vi "DosageCtl.vi"(0 "setpoint volume flow [l/min]":sgl, 1 "pump":bool, 2 "value speed [%]":u8, 3 "shiftReg int":u64, 4 "shiftReg dbl":dbl, 5 "error in (no error)":errorcluster, 6 "setpoint volume [l]":sgl, 7 "value volume flow [l/min]":dbl, 8 "enable":bool, 9 "value volume [dl]":u64, 10 "Actual Start [f]":i64) -> (12 "pump":bool, 14 "speed [%]":dbl, 15 "shiftReg int":u64, 16 "shiftreg dbl":dbl, 17 "enable":bool, 18 "volume[l]":dbl, 19 "error out":errorcluster)   [LabVIEW 2011]
uses:
  <vilib>/functionblocks/Control/PID/PID.vi
  <vilib>/functionblocks/FB Core/FB Core.xnode
  <vilib>/functionblocks/FB Property/FB Overlay DBL.ctl
  <vilib>/functionblocks/NI_FunctionBlock Libraries.lvlib
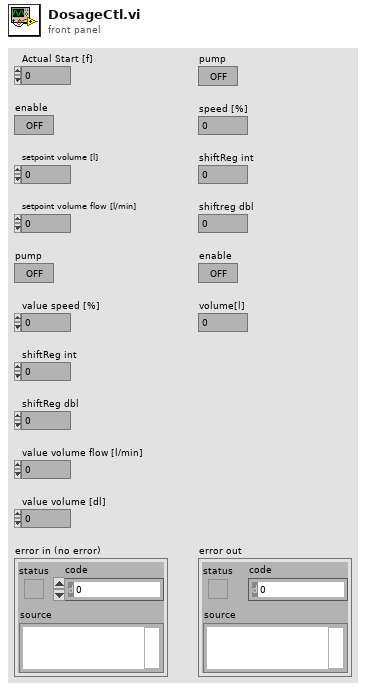
[diagram p1: front panel]
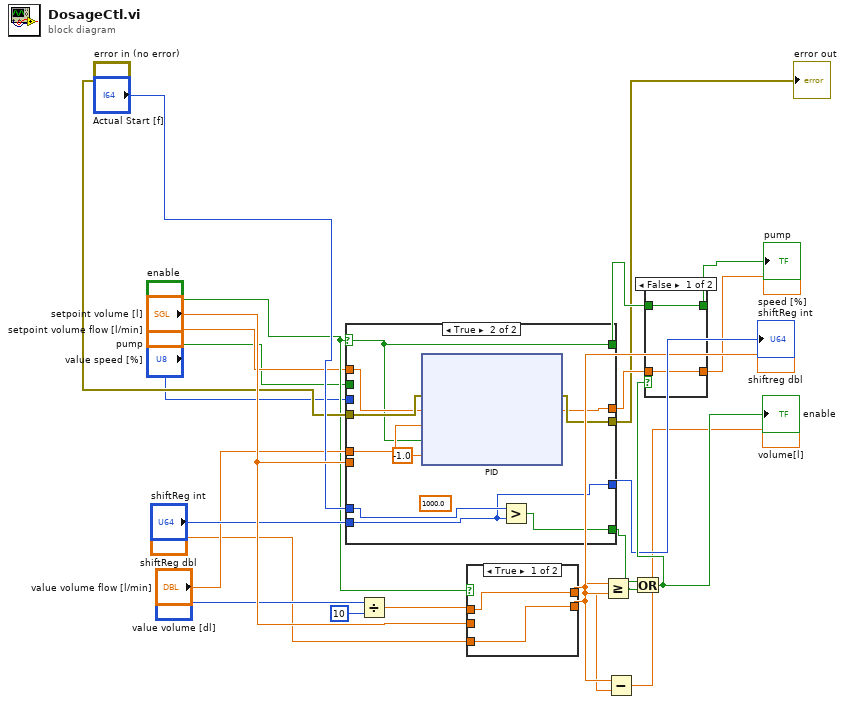
[diagram p0: block diagram]
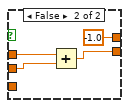
[diagram p2: hidden frame]
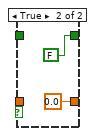
[diagram p3: hidden frame]
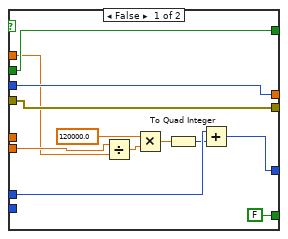
[diagram p4: hidden frame]
diagram:
  n1 = case shown="True" "enable" {
    selector: "enable" -> [_ w42]
    tunnel: [w37 w42] -> w15
    tunnel: "pump" -> [w37 _]
    tunnel: [w36 w45] -> w7
    tunnel: "value speed [%]" -> [w36 _]
    tunnel: [w35 w47] -> w3
    tunnel: "error in (no error)" -> [w35 w46]
    tunnel: "setpoint volume flow [l/min]" -> [w26 w44]
    tunnel: "value volume flow [l/min]" -> [_ w43]
    tunnel: "shiftReg int" -> [_ w39]
    tunnel: "Actual Start [f]" -> [w34 w41]
    tunnel: [w33 w39] -> w21
    tunnel: [FALSE w40] -> w23
    tunnel: "setpoint volume [l]" -> [w27 _]
    frame False {
      n2 = Divide(x=w27, y=w26) -> (x/y=w30:sgl)
      n3 = Multiply(x=120000.0, y=w30) -> (x*y=w31:dbl)
      n4 = To Quad Integer(1:w31) -> (0:w28:i64)
      n5 = Add(x=w34, y=w28) -> (x+y=w33:i64)
    }
    frame True {
      (unwired) 1000.0 ("y")
      n6 = xnode "PID"("error in"=w46, "setpoint"=w44, "process variable"=w43, "auto? (T)"=w42, "dt (s)"=-1.0) -> ("error out"=w47:errorcluster, "output"=w45:dbl)
      n7 = Greater?(x=w41, y=w39) -> (0:w40:bool)
    }
  }
  "shiftReg int" <- w21
  "error out" <- w3
  n8 = Divide(x="value volume [dl]", y=u64 10) -> (x/y=w24:dbl)
  n9 = case shown="True" "enable" {
    tunnel: "setpoint volume [l]" -> [_ w118]
    tunnel: w24 -> [w114 w117]
    tunnel: [w115 w119] -> w12
    tunnel: "shiftReg dbl" -> [w115 _]
    tunnel: [w114 -1.0] -> w11
    frame True {
    }
    frame False {
      n10 = Add(x=w117, y=w118) -> (x+y=w119:dbl)
    }
  }
  "shiftreg dbl" <- w12
  n11 = Greater Or Equal?(x=w11, y=w12) -> (x >= y?=w5:bool)
  n12 = Subtract(x=w12, y=w11) -> (x-y=→"volume[l]":dbl)
  n13 = Or(x=w23, y=w5) -> (x .or. y?=w22:bool)
  "enable" <- w22
  n14 = case shown="False" w22 {
    tunnel: [w121 0.0 ("output")] -> w6
    tunnel: w7 -> [w121 _]
    tunnel: [w120 FALSE ("P-4")] -> w16
    tunnel: w15 -> [w120 _]
    frame False {
    }
    frame True {
    }
  }
  "pump" <- w16
  "speed [%]" <- w6
